vi "Select Dialog.vi"(11 "Item Names":string[](array[string])) -> (0 "Install?":bool, 3 "candidates out":i32[](array[numeric]))   [LabVIEW 2017, in "_Try Beta Version of CSMF.lvlib"]
uses:
  _Try Beta Version of CSMF.lvlib
panel:
  in  "Explore to folder":bool
  in  "Cancel":bool
  in  "Install":bool
  in  "candidates":i32[](listbox)
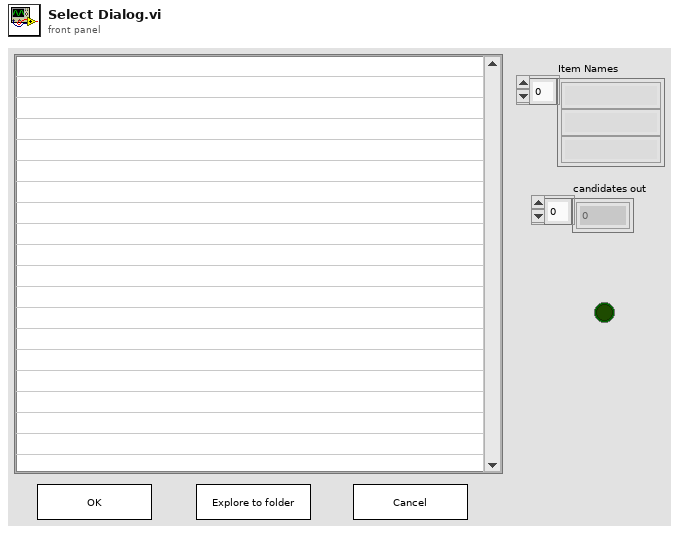
[diagram p1: front panel]
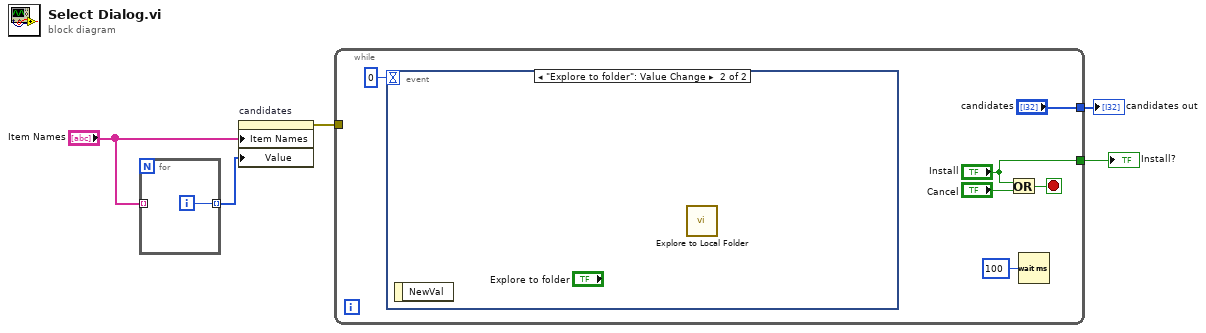
[diagram p0: block diagram]
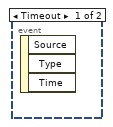
[diagram p2: hidden frame]
diagram:
  n1 = for {
    tunnel: "Item Names" -> [_] mode=indexing
    tunnel: [w6] -> w4 mode=indexing
    i -> [w6]
  }
  n2 = property on="candidates" class="LstBox (strict)"("Item Names"="Item Names", "Value"=w4) -> (error out=w1:errorcluster)  [unwired: 2 in, 1 out]
  n3 = while {
    tunnel: ["Install"] -> w3
    tunnel: ["candidates"] -> w2
    tunnel: w1 -> [_]
    stop <- w11 stop-if-true
    n4 = event shown="[1] \"Explore to folder\": Value Change" {
      selector: _ -> [_ _]
      dyn-events: _ -> [_ _]
      timeout: 0 -> [_ _]
      event Timeout {
        n5 = event-data() -> ()  [unwired: 1 in, 3 out]
      }
      event "Explore to folder": Value Change {
        n6 = event-data() -> ()  [unwired: 1 in, 1 out]
        n7 = call "Explore to Local Folder.vi"() -> ()  [unwired: 11 in, 1 out]
      }
    }
    n8 = Or(x="Install", y="Cancel") -> (x .or. y?=w11:bool)
    n9 = Wait (ms)(milliseconds to wait=u32 100) -> ()  [unwired: 1 out]
  }
  "Install?" <- w3
  "candidates out" <- w2
